vi "Test - Save And Load.vi"   [LabVIEW 2015, in "System Config.lvclass"]
uses:
  System Config.lvclass
  Re-use Libraries/Utility/Utility.lvlib
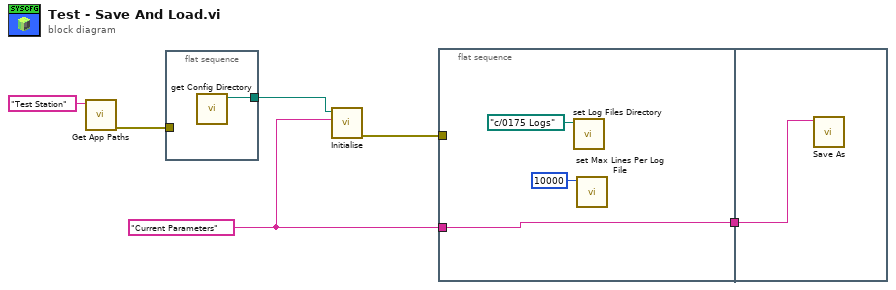
[diagram p0: block diagram]
diagram:
  w3 = "Current Parameters" ("Config Name")
  n1 = call "Get App Paths.vi"("Build Name"="Test Station") -> ("error out"=w2:errorcluster)  [unwired: 9 in, 1 out]
  n2 = flat-sequence {
    tunnel: [w7] -> w6
    tunnel: w2 -> [_]
    frame #0 {
      n3 = call "get Config Directory.vi"() -> ("Config Dir"=w7:path)  [unwired: 11 in]
    }
  }
  n4 = call "Initialise.vi"("Config Name"=w3, "Config Directory"=w6) -> ("error out"=w5:errorcluster)  [unwired: 9 in]
  n5 = flat-sequence {
    tunnel: w5 -> [_]
    tunnel: [w8] -> w4
    tunnel: w3 -> [w8]
    tunnel: w4 -> [w11]
    frame #0 {
      n6 = call "set Log Files Directory.vi"("Log Files Directory"=path "c:/0175 Logs") -> ()  [unwired: 11 in]
      n7 = call "set Max Lines Per Log File.vi"("Max Lines Per Log File"=10000) -> ()  [unwired: 11 in]
    }
    frame #1 {
      n8 = call "Save As.vi"("Config Name"=w11) -> ()  [unwired: 10 in, 1 out]
    }
  }
